vi "Send image to image display controller-subvi.vi"(0 "Image":T1, 1 "Window Title":string, 2 "Window Number":i32, 3 "error in":errorcluster, 4 "Image Type":T2 items=["Grayscale (U8)", "Grayscale (I16)", "Grayscale (SGL)", "Complex (CSG)", "RGB (U32)", "HSL (U32)", "RGB (U64)", "Grayscale (U16)"], 5 "Start display controller?":bool, 6 "Quit display controller?":bool) -> (7 "Image Out":T1, 10 "error out":errorcluster)   [LabVIEW 2014]
doc: "Uses a user event to send an image to Glimpse Image Display controller which is running in a separate thread, if both Start and Quit inputs are false.\n\nStart = TRUE launches the display controller as a separate thread; all other inputs are ignored.\n\nQuit = TRUE sends a message to the controller telling is to close the display windows and quit."
uses:
  <vilib>/vision/Image Controls.llb/IMAQ Image.ctl
  ctt's/Image to Display event.ctt
  Globals/Initilize Globals.vi
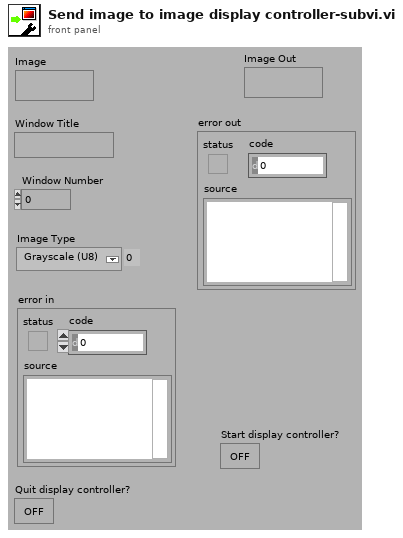
[diagram p1: front panel]
types:
  T1 = typedef "IMAQ Image.ctl" = refnum<image>
  T2 = typedef "Image Type" = u32
  T3 = typedef "Image to Display event.ctt" = cluster{"Image":T1, "Window Title":string, "Window Number":i32, "Image Type":T2, "Quit display controller?":bool}
  T4 = enum32{"Bad", "Idle", "Run top level", "Running"}
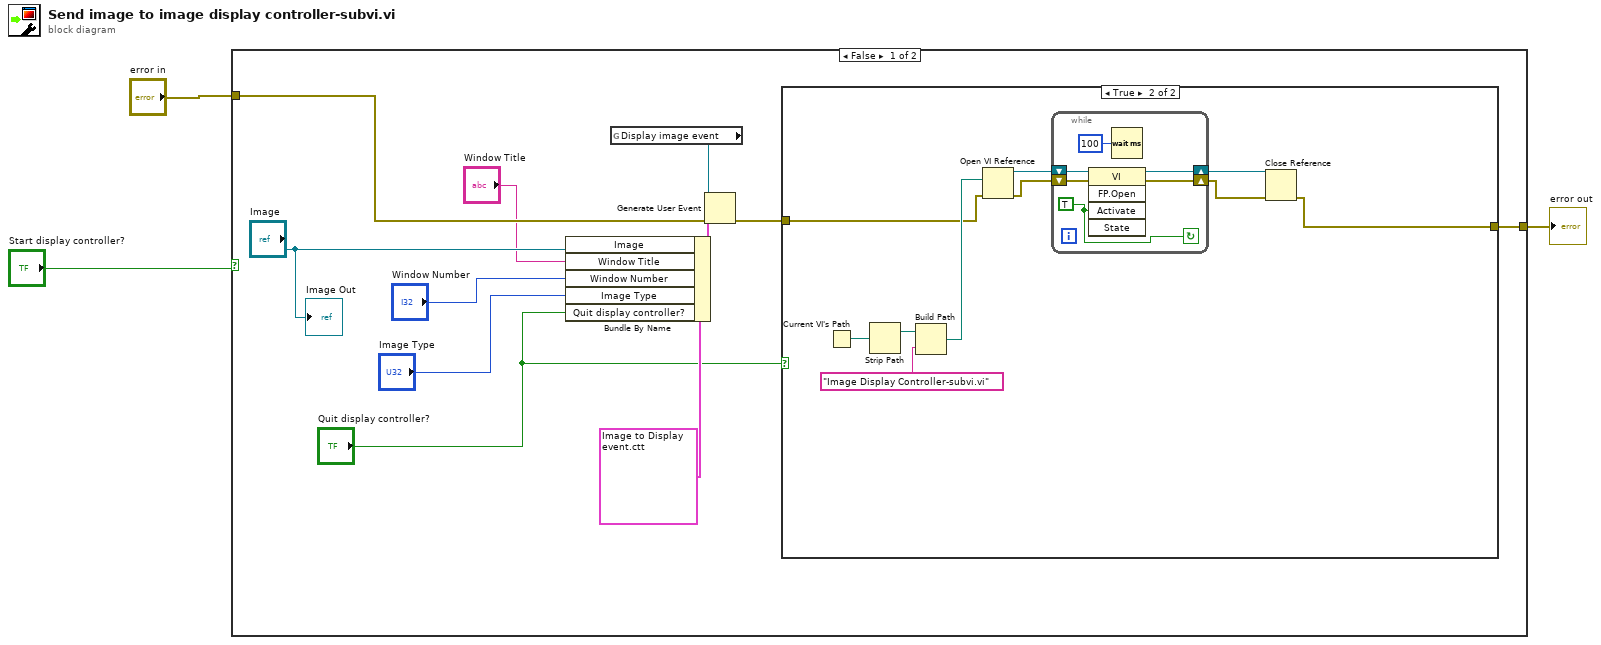
[diagram p0: block diagram]
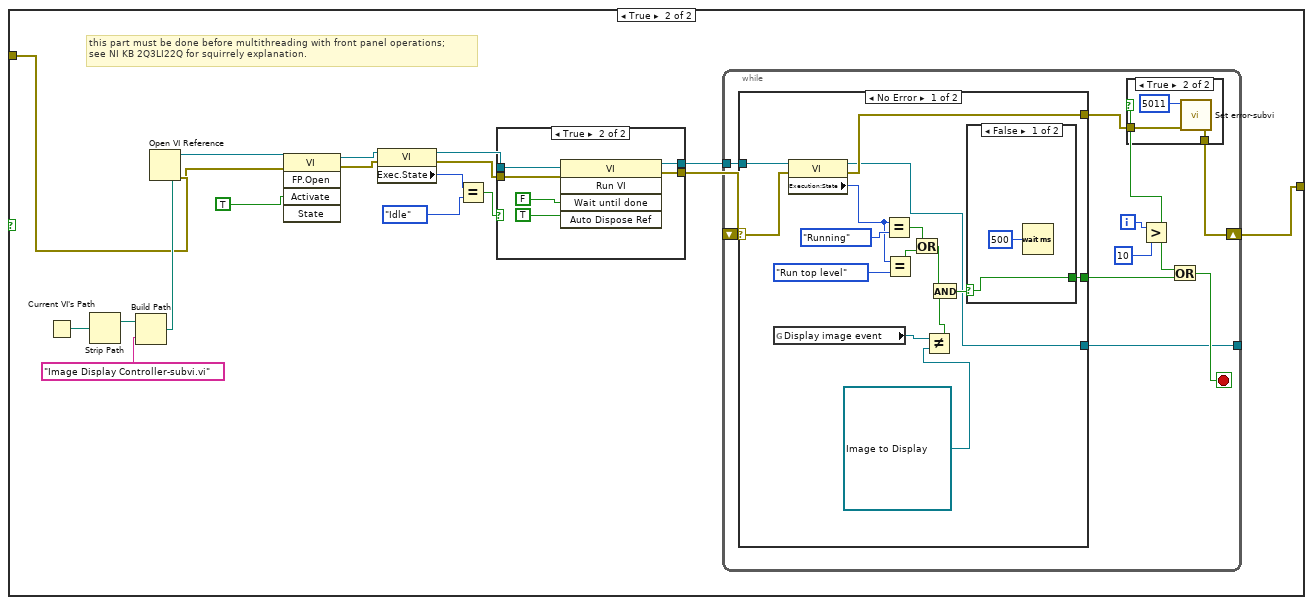
[diagram p3: hidden frame]
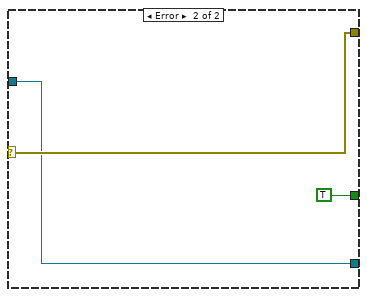
[diagram p7: hidden frame]
diagram:
  n1 = case shown="False" "Start display controller?" {
    tunnel: [w4 w44] -> w3
    tunnel: "error in" -> [w13 w45]
    frame False {
      n2 = Bundle By Name(cluster=T3 {"Image"=refnum, "Window Title"="", "Window Number"=0, "Image Type"=0, "Quit display controller?"=FALSE} ("event data"), "Image"="Image", "Window Title"="Window Title", "Window Number"="Window Number", "Image Type"="Image Type", "Quit display controller?"="Quit display controller?") -> (w10:T3)
      n3 = global read "Initilize Globals.vi" "Display image event"() -> (w12:refnum<user-event>)
      n4 = Generate User Event(user event=w12, event data cluster=w10, error in=w13) -> (error out=w6:errorcluster)  [unwired: 1 in, 1 out]
      n5 = case shown="True" "Quit display controller?" {
        tunnel: w6 -> [w15 w19]
        tunnel: [w15 w16] -> w4
        frame False {
        }
        frame True {
          n6 = Current VI's Path() -> (path=w21:path)
          n7 = Strip Path(path=w21) -> (stripped path=w20:path)  [unwired: 1 out]
          n8 = Build Path(base path=w20, name or relative path="Image Display Controller-subvi.vi") -> (appended path=w23:path)
          n9 = Open VI Reference(vi path=w23, error in (no error)=w19) -> (vi reference=w25:refnum<vi>, error out=w24:errorcluster)  [unwired: 4 out]
          n10 = while {
            shift-right: [w28] -> w18
            shift-left: w25 -> [w30]
            shift-right: [w27] -> w17
            shift-left: w24 -> [w29]
            stop <- w26 continue-if-true
            w26 = TRUE
            n11 = invoke class="VI" method="FP.Open"(reference=w30, error in=w29, "Activate"=w26) -> (reference out=w28:refnum<vi>, error out=w27:errorcluster)  [unwired: 2 in, 3 out]
            n12 = Wait (ms)(milliseconds to wait=u32 100) -> ()  [unwired: 1 out]
          }
          n13 = Close Reference(reference=w18, error in (no error)=w17) -> (error out=w16:errorcluster)
        }
      }
      "Image Out" <- "Image"
    }
    frame True {
      # "this part must be done before multithreading with front panel operations;\nsee NI KB 2Q3LI22Q for squirrely explanation."
      n14 = Current VI's Path() -> (path=w47:path)
      n15 = Strip Path(path=w47) -> (stripped path=w46:path)  [unwired: 1 out]
      n16 = Build Path(base path=w46, name or relative path="Image Display Controller-subvi.vi") -> (appended path=w49:path)
      n17 = Open VI Reference(vi path=w49, error in (no error)=w45) -> (vi reference=w40:refnum<vi>, error out=w41:errorcluster)  [unwired: 4 out]
      n18 = invoke class="VI" method="FP.Open"(reference=w40, error in=w41, "Activate"=TRUE ("Front Panel Window:Open")) -> (reference out=w38:refnum<vi>, error out=w37:errorcluster)  [unwired: 2 in, 3 out]
      n19 = property class="VI"(reference=w38, error in=w37) -> (reference out=w32:refnum<vi>, error out=w33:errorcluster, "Exec.State"=w36:T4)
      n20 = Equal?(x=w36, y=T4."Idle" ("Execution:State")) -> (x = y?=w34:bool)
      n21 = case shown="True" w34 {
        tunnel: [w51 w56] -> w43
        tunnel: [w50 w55] -> w42
        tunnel: w32 -> [w51 w53]
        tunnel: w33 -> [w50 w52]
        frame False {
        }
        frame True {
          n22 = invoke class="VI" method="Run VI"(reference=w53, error in=w52, "Wait until done"=FALSE, "Auto Dispose Ref"=TRUE ("Wait until done")) -> (reference out=w56:refnum<vi>, error out=w55:errorcluster)  [unwired: 1 in, 3 out]
        }
      }
      n23 = while {
        tunnel: w43 -> [w67]
        shift-right: [w60] -> w44
        shift-left: w42 -> [w66]
        tunnel: [w58] -> _
        i -> [w65]
        stop <- w62 stop-if-true
        n24 = case shown="No Error" w66 {
          selector: w66 -> [w75 w91]
          tunnel: w67 -> [w78 w90]
          tunnel: [w76 TRUE] -> w63
          tunnel: [w74 w91] -> w61
          tunnel: [w73 w90] -> w58
          frame No Error {
            n25 = global read "Initilize Globals.vi" "Display image event"() -> (w84:refnum<user-event>)
            n26 = property class="VI"(reference=w78, error in=w75) -> (reference out=w73:refnum<vi>, error out=w74:errorcluster, "Execution:State"=w79:T4)
            n27 = Equal?(x=w79, y=T4."Running" ("Execution:State")) -> (x = y?=w83:bool)
            n28 = Equal?(x=w79, y=T4."Run top level" ("Execution:State")) -> (x = y?=w82:bool)
            n29 = Or(x=w83, y=w82) -> (x .or. y?=w85:bool)
            n30 = Not Equal?(x=w84, y=refnum<user-event> refnum ("Display image event")) -> (x != y?=w86:bool)
            n31 = And(x=w85, y=w86) -> (x .and. y?=w77:bool)
            n32 = case shown="False" w77 {
              selector: w77 -> [w87 w89]
              tunnel: [w87 w89] -> w76
              frame False {
                n33 = Wait (ms)(milliseconds to wait=u32 500) -> ()  [unwired: 1 out]
              }
              frame True {
              }
            }
          }
          frame Error {
          }
        }
        n34 = Greater?(x=w65, y=10) -> (0:w59:bool)
        n35 = case shown="True" w59 {
          tunnel: w61 -> [w68 w70]
          tunnel: [w68 w69] -> w60
          frame False {
          }
          frame True {
            n36 = call "Set error-subvi.vi"("code"=5011, "error in"=w70) -> ("error out"=w69:errorcluster)  [unwired: 6 in]
          }
        }
        n37 = Or(x=w59, y=w63) -> (x .or. y?=w62:bool)
      }
    }
  }
  "error out" <- w3
